vi "Create Image of Different Type.vi"(6 "New Image Type":T1 items=["Grayscale (U8)", "Grayscale (I16)", "Grayscale (SGL)", "Complex (CSG)", "RGB (U32)", "HSL (U32)", "RGB (U64)", "Grayscale (U16)"], 8 "error in (no error)":errorcluster, 9 "Name in":string, 10 "Image Dst":T2, 11 "Image Src":T2) -> (0 "error out":errorcluster, 1 "Name out":string, 2 "Image Dst":T2, 4 "Src Image Type":T1 items=["Grayscale (U8)", "Grayscale (I16)", "Grayscale (SGL)", "Complex (CSG)", "RGB (U32)", "HSL (U32)", "RGB (U64)", "Grayscale (U16)"])   [LabVIEW 2021, in "Image.lvlib"]
doc: "If necessary, creates an <B>Image Dst</B> of the requested type. If <B>Image Dst</B> exists but is not of the requested type, casts it to that type."
uses:
  <vilib>/vision/Image Controls.llb/IMAQ Image.ctl
  Image.lvlib
  Strings/Strings.lvlib
panel:
  out "Message":string
  # "see the AlliGator License on the block diagram (Ctrl+E or Window:Show Block Diagram)"
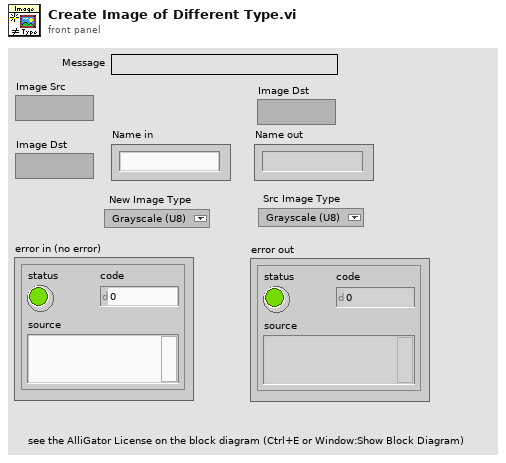
[diagram p1: front panel]
types:
  T1 = typedef "Image Type" = u32
  T2 = typedef "IMAQ Image.ctl" = refnum<image>
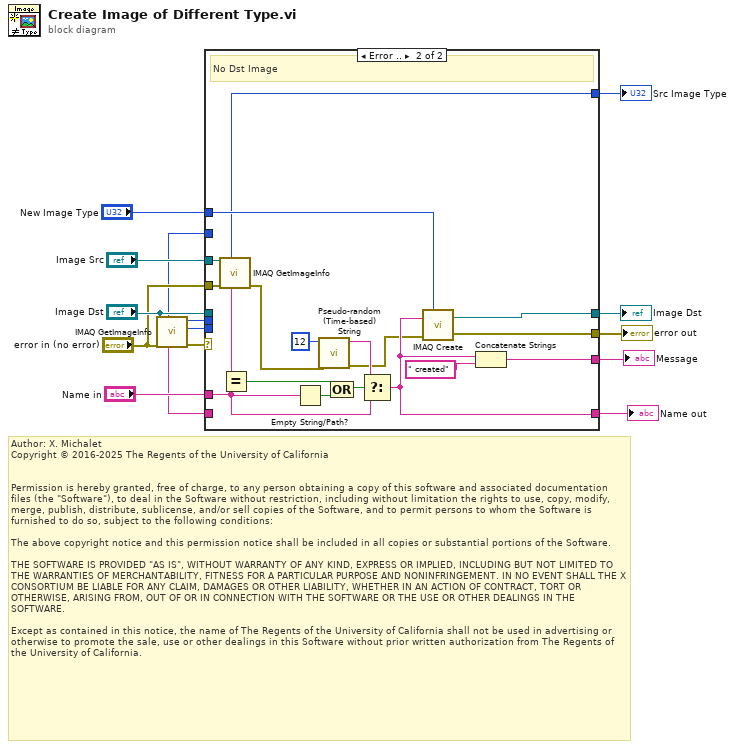
[diagram p0: block diagram]
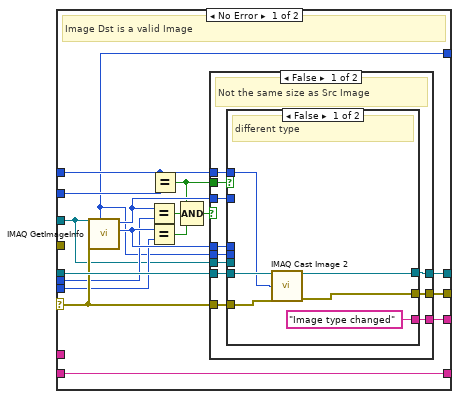
[diagram p2: hidden frame]
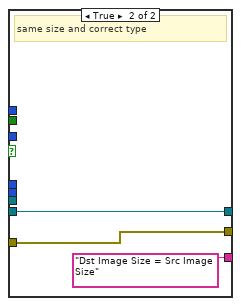
[diagram p4: hidden frame]
diagram:
  # "Author: X. Michalet\nCopyright © 2016-2025 The Regents of the University of California\n \n\nPermission is hereby granted, free of charge, to any person obtaining a copy of this software and associated documentation files (the \"Software\"), to deal in the Software without restriction, including without limitation the rights to use, copy, modify, merge, publish, distribute, sublicense, and/or sell copies of the Software, and to permit persons to whom the Software is furnished to do so, subject to the following conditions:\n\nThe above copyright notice and this permission notice shall be included in all copies or substantial portions of the Software.\n\nTHE SOFTWARE IS PROVIDED \"AS IS\", WITHOUT WARRANTY OF ANY KIND, EXPRESS OR IMPLIED, INCLUDING BUT NOT LIMITED TO THE WARRANTIES OF MERCHANTABILITY, FITNESS FOR A PARTICULAR PURPOSE AND NONINFRINGEMENT. IN NO EVENT SHALL THE X CONSORTIUM BE LIABLE FOR ANY CLAIM, DAMAGES OR OTHER LIABILITY, WHETHER IN AN ACTION OF CONTRACT, TORT OR OTHERWISE, ARISING FROM, OUT OF OR IN CONNECTION WITH THE SOFTWARE OR THE USE OR OTHER DEALINGS IN THE SOFTWARE.\n\nExcept as contained in this notice, the name of The Regents of the University of California shall not be used in advertising or otherwise to promote the sale, use or other dealings in this Software without prior written authorization from The Regents of the University of California."
  n1 = call "IMAQ GetImageInfo"("error in (no error)"="error in (no error)", "Image"="Image Dst") -> ("error out"=w8:errorcluster, "Y Resolution"=w7:i32, "X Resolution"=w6:i32, "Image Name"=w5:string, "Image Type"=w3:T1)  [unwired: 2 in, 3 out]
  n2 = case shown="Error .." w8 {
    selector: w8 -> [w24 _]
    tunnel: "Image Src" -> [w20 w73]
    tunnel: "Name in" -> [_ w67]
    tunnel: [w28 w57] -> w13
    tunnel: [w19 w72] -> w12
    tunnel: [w29 w68] -> w11
    tunnel: "Image Dst" -> [w30 _]
    tunnel: [w25 w70] -> w10
    tunnel: w7 -> [w23 _]
    tunnel: w6 -> [w22 _]
    tunnel: w3 -> [w18 _]
    tunnel: w5 -> [w19 _]
    tunnel: "error in (no error)" -> [_ w63]
    tunnel: "New Image Type" -> [w17 w58]
    tunnel: [w16 w56] -> w1
    frame No Error {
      # "Image Dst is a valid Image"
      n3 = call "IMAQ GetImageInfo"("error in (no error)"=w24, "Image"=w20) -> ("Y Resolution"=w26:i32, "X Resolution"=w27:i32, "Image Type"=w16:T1)  [unwired: 2 in, 5 out]
      n4 = Equal?(x=w27, y=w22) -> (x = y?=w33:bool)
      n5 = Equal?(x=w26, y=w23) -> (x = y?=w32:bool)
      n6 = Equal?(x=w17, y=w18) -> (x = y?=w21:bool)
      n7 = Compound Arithmetic op=AND(w21, w33, w32) -> (w31:bool)
      n8 = case shown="False" w31 {
        tunnel: w30 -> [w44 w55]
        tunnel: [w43 w55] -> w29
        tunnel: [w42 w53] -> w28
        tunnel: w27 -> [w41 _]
        tunnel: w26 -> [w40 _]
        tunnel: w24 -> [w39 w53]
        tunnel: [w38 "Dst Image Size = Src Image Size"] -> w25
        tunnel: w21 -> [w37 _]
        tunnel: w20 -> [w36 _]
        tunnel: w16 -> [w35 _]
        tunnel: w17 -> [w34 _]
        frame False {
          # "Not the same size as Src Image"
          n9 = case shown="False" w37 {
            tunnel: w44 -> [w49 w52]
            tunnel: [w45 w52] -> w43
            tunnel: [w46 w51] -> w42
            tunnel: w41 -> [_ _]
            tunnel: w40 -> [_ _]
            tunnel: w39 -> [w47 w51]
            tunnel: ["Image type changed" _] -> w38
            tunnel: w36 -> [_ _]
            tunnel: w35 -> [_ _]
            tunnel: w34 -> [w48 _]
            frame False {
              # "different type"
              n10 = call "IMAQ Cast Image 2"("Image Src"=w49, "Image Type"=w48, "error in (no error)"=w47) -> ("Image Dst Out"=w45:T2, "error out"=w46:errorcluster)  [unwired: 11 in]
            }
            frame True {
              # "Correct type image"
            }
          }
        }
        frame True {
          # "same size and correct type"
        }
      }
    }
    frame Error {
      # "No Dst Image"
      n11 = call "IMAQ GetImageInfo"("error in (no error)"=w63, "Image"=w73) -> ("error out"=w61:errorcluster, "Image Name"=w66:string, "Image Type"=w56:T1)  [unwired: 2 in, 5 out]
      n12 = Equal?(x=w66, y=w67) -> (x = y?=w65:bool)
      n13 = Empty String/Path?(string/path=w67) -> (empty?=w64:bool)
      n14 = call "Pseudo-random (Time-based) String.vi"("Error In"=w61, "Length (10)"=u32 12) -> ("Error Out"=w60:errorcluster, "result string"=w62:string)  [unwired: 8 in]
      n15 = Compound Arithmetic op=OR(w65, w64) -> (w69:bool)
      n16 = Select(t=w62, s=w69, f=w67) -> (s? t:f=w72:string)
      n17 = call "IMAQ Create"("Image Name"=w72, "Image Type"=w58, "error in (no error)"=w60) -> ("New Image"=w68:T2, "error out"=w57:errorcluster)  [unwired: 2 in]
      n18 = Concatenate Strings(w72, " created" ("string")) -> (w70:string)
    }
  }
  "error out" <- w13
  "Image Dst" <- w11
  "Name out" <- w12
  "Message" <- w10
  "Src Image Type" <- w1
